vi "Update 3D Object Position.vi"(8 "error in (no error)":errorcluster, 10 "New Rigid Body Position":T5, 11 "Frame Grabber Data in":T1={"Camera Session"="", "Frame"=refnum, "AVI Refnum"=refnum, "Codecs"=[], "Frame number"=0, "Tracking File Refnum"=refnum, "Tick Count"=0, "Probe Object"=refnum, "Playback Probe Data"=[], "Rigid Body"={"Position"={"x (mm)"=0.0, "y (mm)"=0.0, "z (mm)"=0.0}, "Orientation"={"Pitch (rad)"=0.0, "Yaw (rad)"=0.0, "Roll (rad)"=0.0}, "Quaternion"={"qx"=0.0, "qy"=0.0, "qz"=0.0, "qw"=0.0}, "Tracked?"=FALSE}, "Total no frames playback"=0, "Video FPS"=0.0, "Camera connected?"=FALSE, "Scene"=refnum, "Cropped Frame"=refnum, "Tracker FPS"=0.0, "Crop ROI"=[], "Presentation Values"=[], "Elapsed time (ms)"=0, "Camera frames playback"=0, "Refnums"={"Live Refnum"=refnum, "Record Refnum"=refnum, "Recording Settings Refnum"=refnum, "Playback Refnum"=refnum, "Frame Slider Refnum"=refnum, "Pause Refnum"=refnum, "Home Refnum"=refnum, "Crop Refnum"=refnum, "Clear Crop Refnum"=refnum, "stop refnum"=refnum, "Playback Rate Refnum"=refnum, "Operator Settings Refnums"=refnum, "Presentation Refnum"=refnum, "Gestation Refnum"=refnum, "Crop Time Frame Slider Refnum"=refnum, "Cancel Save Refnum"=refnum, "Reverse Playback Refnum"=refnum, "Connection Settings Refnum"=refnum}, "Dimensions"={"Probe Dimensions"={"Probe Width"=0.0, "Probe Depth"=1.0, "Probe Height"=0.0}, "Room Dimensions"={"Room Width"=0.0, "Room Depth"=0.0, "Room Height"=0.0}}, "Playback Data As Strings"=[], "Cropped Tracking File Refnum"=refnum, "Cropped AVI Refnum"=refnum, "Header"=[], "Total euclidian distance"=0.0, "Annotation File Path"=path "", "Playback File Path"=path ""}) -> (0 "error out":errorcluster, 3 "Frame Grabber Data out":T1={"Camera Session"="", "Frame"=refnum, "AVI Refnum"=refnum, "Codecs"=[], "Frame number"=0, "Tracking File Refnum"=refnum, "Tick Count"=0, "Probe Object"=refnum, "Playback Probe Data"=[], "Rigid Body"={"Position"={"x (mm)"=0.0, "y (mm)"=0.0, "z (mm)"=0.0}, "Orientation"={"Pitch (rad)"=0.0, "Yaw (rad)"=0.0, "Roll (rad)"=0.0}, "Quaternion"={"qx"=0.0, "qy"=0.0, "qz"=0.0, "qw"=0.0}, "Tracked?"=FALSE}, "Total no frames playback"=0, "Video FPS"=0.0, "Camera connected?"=FALSE, "Scene"=refnum, "Cropped Frame"=refnum, "Tracker FPS"=0.0, "Crop ROI"=[], "Presentation Values"=[], "Elapsed time (ms)"=0, "Camera frames playback"=0, "Refnums"={"Live Refnum"=refnum, "Record Refnum"=refnum, "Recording Settings Refnum"=refnum, "Playback Refnum"=refnum, "Frame Slider Refnum"=refnum, "Pause Refnum"=refnum, "Home Refnum"=refnum, "Crop Refnum"=refnum, "Clear Crop Refnum"=refnum, "stop refnum"=refnum, "Playback Rate Refnum"=refnum, "Operator Settings Refnums"=refnum, "Presentation Refnum"=refnum, "Gestation Refnum"=refnum, "Crop Time Frame Slider Refnum"=refnum, "Cancel Save Refnum"=refnum, "Reverse Playback Refnum"=refnum, "Connection Settings Refnum"=refnum}, "Dimensions"={"Probe Dimensions"={"Probe Width"=0.0, "Probe Depth"=1.0, "Probe Height"=0.0}, "Room Dimensions"={"Room Width"=0.0, "Room Depth"=0.0, "Room Height"=0.0}}, "Playback Data As Strings"=[], "Cropped Tracking File Refnum"=refnum, "Cropped AVI Refnum"=refnum, "Header"=[], "Total euclidian distance"=0.0, "Annotation File Path"=path "", "Playback File Path"=path ""})   [LabVIEW 2017]
uses:
  Controls/Rigid Body Info.ctl
  Controls/Position.ctl
  Controls/Orientation.ctl
  Controls/Frame Grabber Data.ctl
  <vilib>/userdefined/High Color/IMAQdx.ctl
  <vilib>/vision/Image Controls.llb/IMAQ Image.ctl
  <vilib>/vision/Avi.llb/IMAQ AVI2 Refnum.ctl
  Controls/Refnums.ctl
  Controls/Recording Settings.ctl
  Controls/Operator Settings.ctl
  Controls/Operator.ctl
  Controls/Connection Settings.ctl
  Controls/Tracker Type.ctl
  Controls/COM Port.ctl
  Controls/Dimensions.ctl
  Controls/Room Dimensions.ctl
  <vilib>/Analysis/baseanly.llb/Real A x B.vi
  <vilib>/Analysis/_algsub.llb/Vector Norm.vi
  <vilib>/Analysis/_algsub.llb/Real Vector Norm.vi
  <vilib>/Analysis/baseanly.llb/Outer Product.vi
  <vilib>/Analysis/baseanly.llb/Real Outer Product.vi
  <vilib>/robotics/Kinematics/Create Lie Group Matrix.vi
  <vilib>/Analysis/Matrix/Numeric/Multiply/Multiply.vi
  <vilib>/Analysis/Matrix/Numeric/Multiply/Multiply - RM,R.vi
  <vilib>/Analysis/Matrix/Numeric/Multiply/Multiply - R,RM.vi
  <vilib>/Analysis/Matrix/Numeric/Add/Add.vi
  <vilib>/Analysis/Matrix/Numeric/Add/Add - RM,RM.vi
  <vilib>/Analysis/baseanly.llb/Real Inverse Matrix.vi
  <vilib>/picture/3D Picture Control/NI_3D Picture Control.lvlib
  <vilib>/robotics/Kinematics/NI_Kinematics.lvlib
  <vilib>/Analysis/NI_AALBase.lvlib
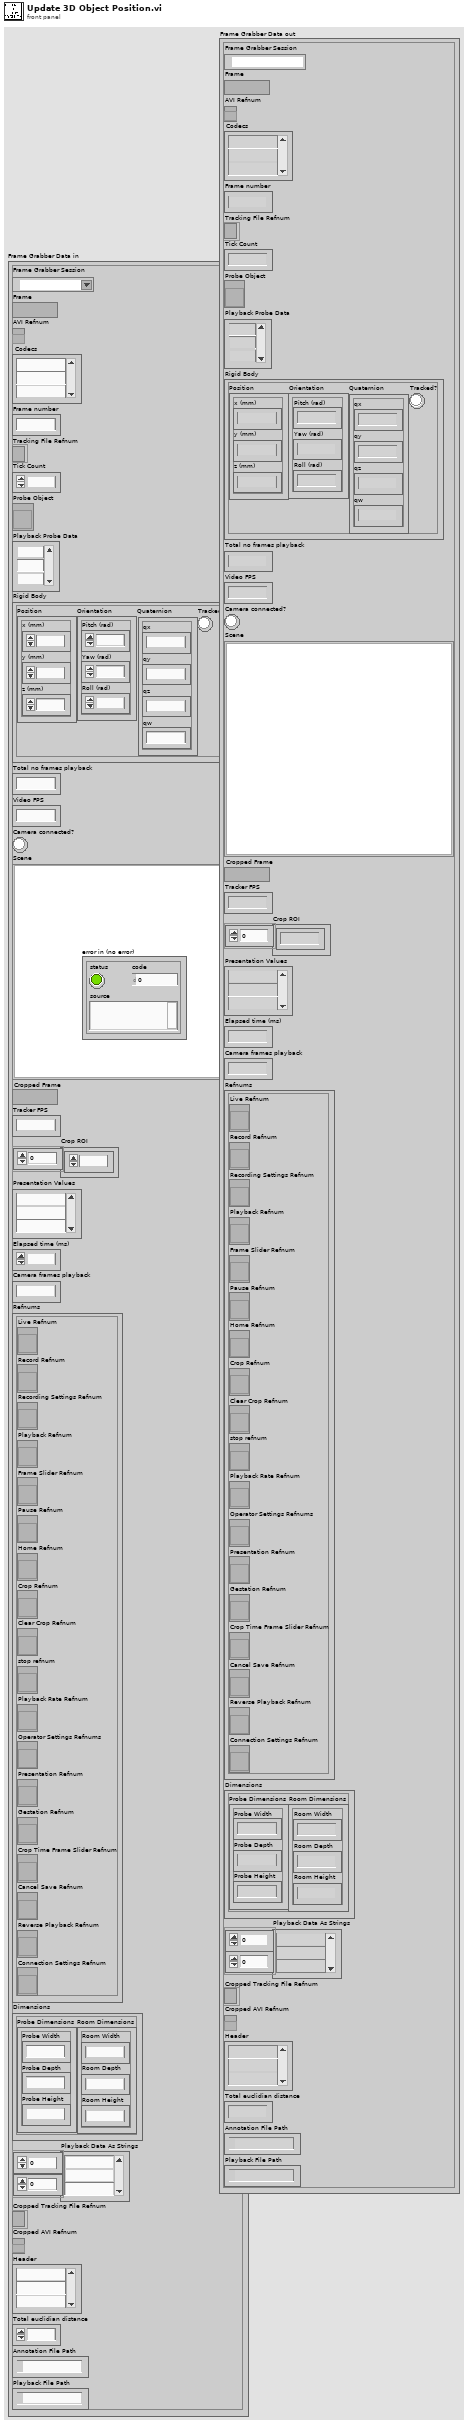
[diagram p1: front panel]
types:
  T1 = typedef "Frame Grabber Data.ctl" = cluster{"Camera Session":T2, "Frame":T3, "AVI Refnum":T4, "Codecs":string[], "Frame number":u32, "Tracking File Refnum":refnum<file>, "Tick Count":u32, "Probe Object":refnum<vi>, "Playback Probe Data":dbl[][], "Rigid Body":T5, "Total no frames playback":i32, "Video FPS":dbl, "Camera connected?":bool, "Scene":refnum<vi>, "Cropped Frame":T3, "Tracker FPS":dbl, "Crop ROI":i32[], "Presentation Values":string[], "Elapsed time (ms)":u32, "Camera frames playback":u32, "Refnums":T8, "Dimensions":T9, "Playback Data As Strings":string[][], "Cropped Tracking File Refnum":refnum<file>, "Cropped AVI Refnum":T4, "Header":string[], "Total euclidian distance":dbl, "Annotation File Path":path, "Playback File Path":path}
  T2 = typedef "IMAQdx.ctl" = refnum<k21>
  T3 = typedef "IMAQ Image.ctl" = refnum<image>
  T4 = typedef "IMAQ AVI2 Refnum.ctl" = refnum<k20>
  T5 = typedef "Rigid Body Info.ctl" = cluster{"Position":T6, "Orientation":T7, "Quaternion":cluster{"qx":sgl, "qy":sgl, "qz":sgl, "qw":sgl}, "Tracked?":bool}
  T6 = typedef "Position.ctl" = cluster{"x (mm)":sgl, "y (mm)":sgl, "z (mm)":sgl}
  T7 = typedef "Orientation.ctl" = cluster{"Pitch (rad)":sgl, "Yaw (rad)":sgl, "Roll (rad)":sgl}
  T8 = typedef "Refnums.ctl" = cluster{"Live Refnum":refnum<vi>, "Record Refnum":refnum<vi>, "Recording Settings Refnum":refnum<vi>, "Playback Refnum":refnum<vi>, "Frame Slider Refnum":refnum<vi>, "Pause Refnum":refnum<vi>, "Home Refnum":refnum<vi>, "Crop Refnum":refnum<vi>, "Clear Crop Refnum":refnum<vi>, "stop refnum":refnum<vi>, "Playback Rate Refnum":refnum<vi>, "Operator Settings Refnums":refnum<vi>, "Presentation Refnum":refnum<vi>, "Gestation Refnum":refnum<vi>, "Crop Time Frame Slider Refnum":refnum<vi>, "Cancel Save Refnum":refnum<vi>, "Reverse Playback Refnum":refnum<vi>, "Connection Settings Refnum":refnum<vi>}
  T9 = typedef "Dimensions.ctl" = cluster{"Probe Dimensions":cluster{"Probe Width":sgl, "Probe Depth":sgl, "Probe Height":sgl}, "Room Dimensions":T10}
  T10 = typedef "Room Dimensions.ctl" = cluster{"Room Width":dbl, "Room Depth":dbl, "Room Height":dbl}
  T11 = typedef "NI_Kinematics.lvlib/Quaternion.ctl" = dbl[]
  T12 = typedef "NI_Matrix.lvlib/RealMatrix.ctl" = dbl[][]
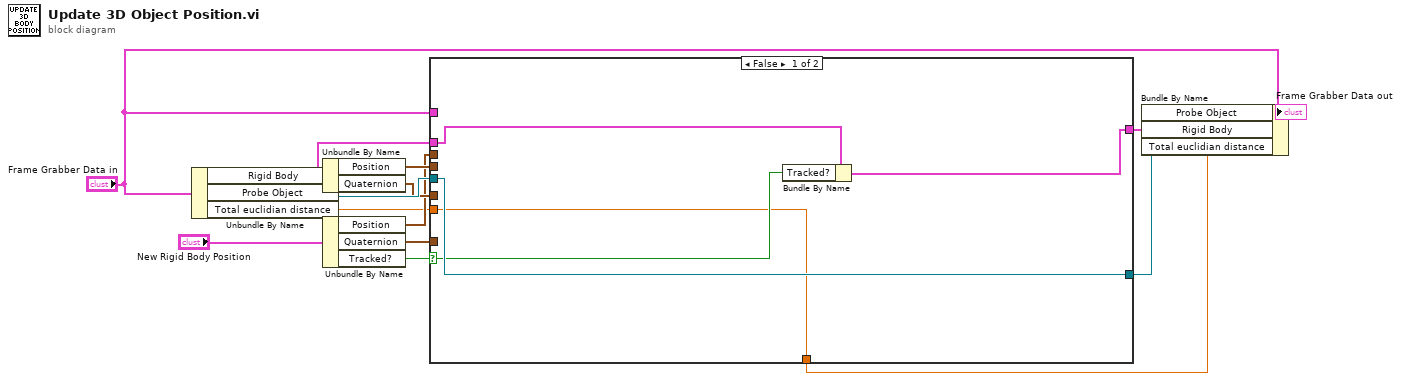
[diagram p0: block diagram]
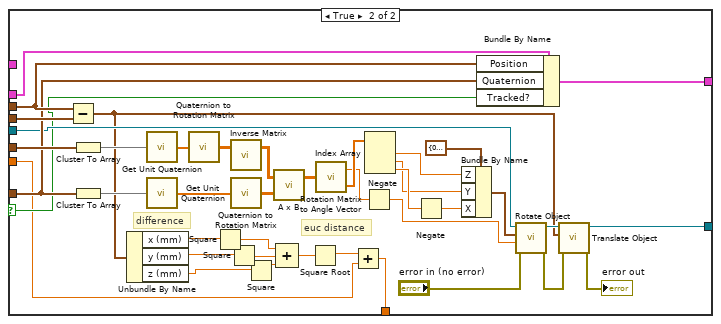
[diagram p2: hidden frame]
diagram:
  n1 = Unbundle By Name("Frame Grabber Data in") -> ("Rigid Body"=w9:T5, "Probe Object"=w14:refnum<vi>, "Total euclidian distance"=w2:dbl)
  n2 = Unbundle By Name(w9) -> ("Position"=w12:T6, "Quaternion"=w10:cluster{"qx":sgl, "qy":sgl, "qz":sgl, "qw":sgl})
  n3 = Unbundle By Name("New Rigid Body Position") -> ("Position"=w8:T6, "Quaternion"=w7:cluster{"qx":sgl, "qy":sgl, "qz":sgl, "qw":sgl}, "Tracked?"=w6:bool)
  n4 = case shown="False" w6 {
    selector: w6 -> [w16 w33]
    tunnel: w14 -> [w19 w44]
    tunnel: "Frame Grabber Data in" -> [_ _]
    tunnel: w12 -> [_ w58]
    tunnel: w10 -> [_ w57]
    tunnel: w9 -> [w18 w56]
    tunnel: w8 -> [_ w55]
    tunnel: w7 -> [_ w54]
    tunnel: [w19 w32] -> w5
    tunnel: [w17 w31] -> w4
    tunnel: w2 -> [w15 w21]
    tunnel: [w15 w20] -> w1
    frame False {
      n5 = Bundle By Name(cluster=w18, "Tracked?"=w16) -> (w17:T5)
    }
    frame True {
      # "euc distance"
      # "difference"
      n6 = Subtract(x=w55, y=w58) -> (x-y=w30:T6)
      n7 = Cluster To Array(cluster=w57) -> (array=w38:sgl[])
      n8 = Cluster To Array(cluster=w54) -> (array=w40:sgl[])
      n9 = Unbundle By Name(w30) -> ("x (mm)"=w29:sgl, "y (mm)"=w28:sgl, "z (mm)"=w27:sgl)
      n10 = call <vilib>:"Get Unit Quaternion.vi"("quaternion"=w38) -> ("unit quaternion"=w37:T11)
      n11 = call <vilib>:"Get Unit Quaternion.vi"("quaternion"=w40) -> ("unit quaternion"=w39:T11)
      n12 = call <vilib>:"Quaternion to Rotation Matrix.vi"("quaternion"=w37) -> ("rotation matrix"=w48:T12)
      n13 = Square(x=w29) -> (x^2=w26:sgl)
      n14 = Square(x=w28) -> (x^2=w25:sgl)
      n15 = call-poly <vilib>:"Inverse Matrix.vi"("Input Matrix"=w48) -> ("Inverse Matrix"=w47:T12)  [unwired: 1 in, 1 out]
      n16 = call <vilib>:"Quaternion to Rotation Matrix.vi"("quaternion"=w39) -> ("rotation matrix"=w46:T12)
      n17 = Square(x=w27) -> (x^2=w24:sgl)
      n18 = call-poly <vilib>:"A x B.vi"("B"=w46, "A"=w47) -> ("A x B"=w49:T12)  [unwired: 1 out]
      n19 = Compound Arithmetic op=ADD(w26, w25, w24) -> (w23:sgl)
      n20 = Square Root(x=w23) -> (sqrt(x)=w22:sgl)
      n21 = call <vilib>:"Rotation Matrix to Angle Vector.vi"("rotation matrix"=w49) -> ("angle"=w50:dbl, "vector"=w53:dbl[])
      n22 = Add(x=w22, y=w21) -> (x+y=w20:dbl)
      n23 = Negate(x=w50) -> (-x=w36:dbl)
      n24 = Index Array(array=w53) -> (element #1=w51:dbl, element #2=w35:dbl, element #3=w52:dbl)  [unwired: 3 in]
      n25 = Negate(x=w52) -> (-x=w34:dbl)
      n26 = Bundle By Name(cluster=cluster{"X":sgl, "Y":sgl, "Z":sgl} {"X"=0.0, "Y"=0.0, "Z"=0.0} ("Axis"), "Z"=w51, "Y"=w35, "X"=w34) -> (w60:cluster{"X":sgl, "Y":sgl, "Z":sgl})
      n27 = Bundle By Name(cluster=w56, "Position"=w55, "Quaternion"=w54, "Tracked?"=w33) -> (w31:T5)
      n28 = call <vilib>:"Rotate Object.vi"("error in (no error)"="error in (no error)", "Angle"=w36, "Axis"=w60, "Scene.Object In"=w44) -> ("error out"=w41:errorcluster, "Scene.Object Out"=w43:refnum<vi>)  [unwired: 6 in]
      n29 = call <vilib>:"Translate Object.vi"("error in (no error)"=w41, "Translation"=w30, "Scene.Object In"=w43) -> ("error out"=→"error out":errorcluster, "Scene.Object Out"=w32:refnum<vi>)  [unwired: 7 in]
    }
  }
  n30 = Bundle By Name(cluster="Frame Grabber Data in", "Probe Object"=w5, "Rigid Body"=w4, "Total euclidian distance"=w1) -> (→"Frame Grabber Data out":T1)
